vi "Group THD and Subgroup THD.vi"   [LabVIEW 2014, in "NI_EP_Power Quality.lvlib"]
doc: "Calculates group total harmonic distortion and subgroup total harmonic distortion, in percentage, according to IEC 61000-4-7:2009. You must manually select the polymorphic instance to use.\n\nThis VI supports measuring single-line and multiple-line systems."
uses:
  <vilib>/addons/Electrical Power/PQ/NI_EP_Power Quality.lvlib
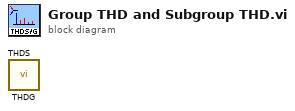
[diagram p0: block diagram]
diagram:
  n1 = call <vilib>:"THDG.vi"() -> ()  [unwired: 9 in, 3 out]
  n2 = call <vilib>:"THDS.vi"() -> ()  [unwired: 9 in, 3 out]
